vi "09_1.vi"() -> ()   [LabVIEW 2018]
panel:
  in  "length":i32=25
  out "Numeric":dbl=25918798.0
  in  "#Elements":i32=2
  in  "Input":string="14\n9\n43\n18\n13\n24\n3\n38\n33\n8\n41\n4\n32\n15\n31\n44\n17\n34\n21\n10\n50\n37\n2\n23\n6\n47\n5\n9\n11\n16\n12\n18\n7\n13\n26\n14\n19\n8\n20\n15\n29\n58\n17\n22\n21\n24\n25\n10\n27\n31\n33\n23\n28\n30\n34\n32\n35\n38\n49\n18\n26\n36\n37\n47\n39\n56\n40\n42\n43\n41\n44\n45\n46\n48\n50\n51\n53\n79\n73\n69\n117\n54\n55\n90\n57\n62\n75\n114\n85\n94\n110\n81\n98\n153\n86\n89\n204\n96\n101\n103\n104\n152\n169\n124\n135\n109\n143\n171\n119\n132\n137\n207\n166\n167\n184\n185\n170\n175\n182\n187\n190\n197\n233\n204\n212\n244\n299\n228\n339\n241\n246\n269\n415\n319\n298\n349\n337\n333\n444\n357\n345\n362\n365\n562\n377\n387\n401\n416\n541\n469\n472\n474\n647\n591\n487\n515\n567\n617\n686\n1158\n793\n670\n678\n702\n864\n710\n856\n781\n817\n764\n1251\n1214\n885\n941\n943\n..."
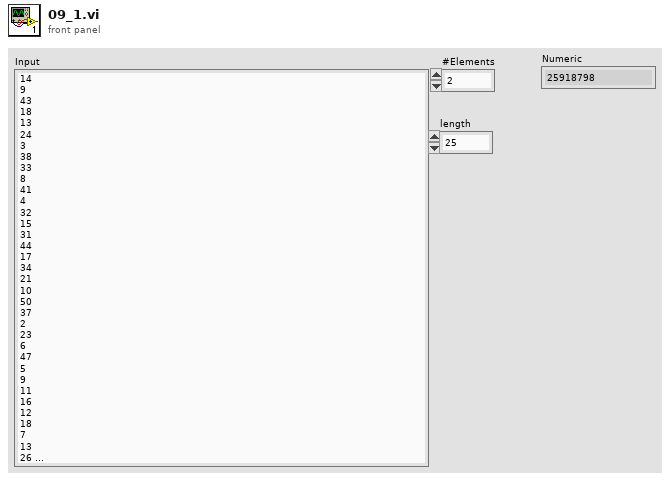
[diagram p1: front panel]
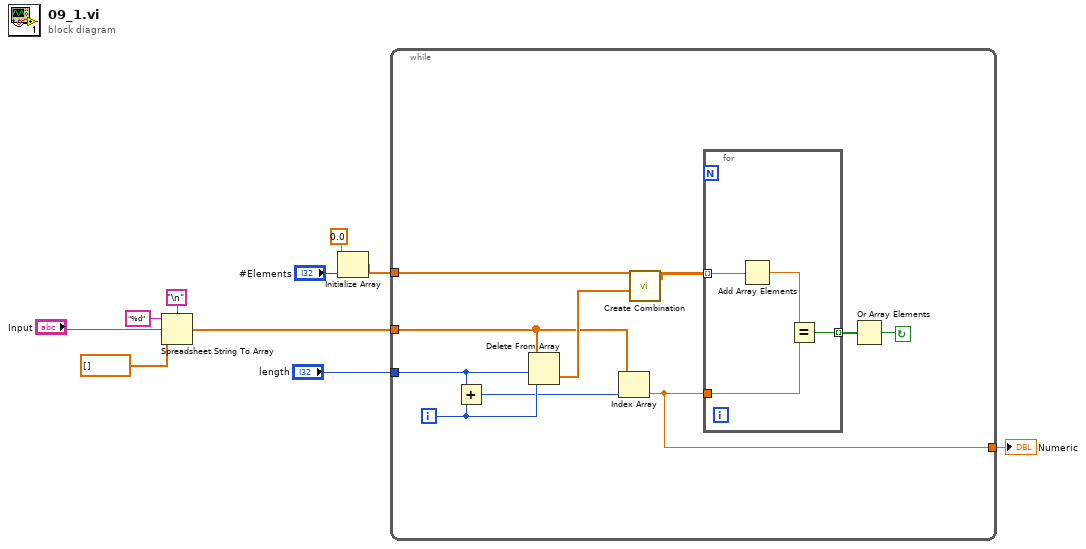
[diagram p0: block diagram]
diagram:
  n1 = Spreadsheet String To Array(delimiter (Tab)="\n", format string="%d", spreadsheet string="Input", array type (2D Dbl)=dbl[] []) -> (array=w3:dbl[])
  n2 = Initialize Array(0.0, "#Elements") -> (w4:dbl[])
  n3 = while {
    tunnel: w4 -> [w20]
    tunnel: w3 -> [w11]
    tunnel: "length" -> [w13]
    tunnel: [w16] -> w1
    i -> [w14]
    stop <- w17 continue-if-true
    n4 = Add(x=w13, y=w14) -> (x+y=w12:i32)
    n5 = Delete From Array(array=w11, length=w13, index=w14) -> (deleted portion=w15:dbl[])  [unwired: 1 out]
    n6 = Index Array(array=w11, index=w12) -> (element=w16:dbl)
    n7 = call "Create Combination.vi"("Array"=w15, "Temp Combination"=w20) -> ("Combinations Out"=w19:dbl[][])  [unwired: 9 in]
    n8 = for {
      tunnel: w19 -> [w24] mode=indexing
      tunnel: w16 -> [w22]
      tunnel: [w21] -> w18 mode=indexing
      n9 = Add Array Elements(numeric array=w24) -> (sum=w23:dbl)
      n10 = Equal?(x=w23, y=w22) -> (x = y?=w21:bool)
    }
    n11 = Or Array Elements(Boolean array=w18) -> (logical OR=w17:bool)
  }
  "Numeric" <- w1
